vi "Begin.vi"(8 "error in":errorcluster) -> (0 "error out":errorcluster)   [LabVIEW 2019]
doc: "Called before other user functions, this VI is expected to open initial I/O refnums, load in file data, and do all program initialization. Notice that the <B>error out</B> terminal is simply used for data flow. Wiring it to other structures or subVIs ensures that this VI runs first."
uses:
  <vilib>/Rock Robotics/SystemInterfaces/DIO/FPGA_DIOPWMChannel.ctl
  <vilib>/Rock Robotics/WPI/SafetyOutput/WPI_SafetyOutputConfigMenu.ctl
  <vilib>/Rock Robotics/WPI/DriverStation/WPI_DriverStationRobotMode2.ctl
  <vilib>/Rock Robotics/WPI/Joystick/WPI_JoystickDeviceEnum.ctl
  <vilib>/Rock Robotics/SystemInterfaces/AI/FPGA_AIGyroChannel.ctl
  <vilib>/Rock Robotics/SystemInterfaces/DIO/FPGA_DIOChannel.ctl
  <vilib>/Rock Robotics/WPI/Encoder/WPI_EncoderType.ctl
  <vilib>/Rock Robotics/WPI/RobotDrive/WPI_RobotDriveOpen2MotorWithTalon.vi
  Robot Global Data.vi
  <vilib>/Rock Robotics/Network Tables/NT Write String Array.vi
  <vilib>/Rock Robotics/WPI/Gyro/WPI_GyroAnalogOpen.vi
  <vilib>/Rock Robotics/WPI/Counter/WPI_CounterDigitalInputToDigitalSource.vi
panel:
  in  "Tab Control":T1(tab)
  # "Instructions:\nThis should create a path, show the data on the various tabs and optionally write the motor demands and expected results to a file for use on a a robot..\n1) Enter robot data on Robot Data Tab\n2) Define your path definitions.\n3) Define the time increment.  0.020 is chosen since that matches the normal loop time.\n4) Press calculate path.  If a good path was calculated it will be displayed on the Tank Data tab, and the Ready to Execute will indicate execution can begin.\nThe path can be recalculated many times before selecting execute.\n\nTo write to a file.\n5) Select the file name\n6) This example uses \"steps\", sequential numbers for inclusion into a list based autonomous routine.  Including the step number if optional.\n7) This uses command numbers to indicate first, last, and intermediate steps.  This allows some simplification of the execution routine.  It\nalso allows the path to be executed backwards if desired.  The command numbers are changeable.\n8) Press \"Create Command List\".\n\nNotes:\n- PC robot simulataion is disabled in this program.  The code is still there if you want to restore it and try it out.  Use one of the other test programs \nto simulate the path on a PC.\n- The path generation logic doesn't account distribution of speed to the left and right wheels.  As a result the maximum speed can be exceeded.\nIf this happens, but Path Speed > Max light will light and Ready to Execute will not light.  Lower the maximum speed in the Robot Data tab\nand recalulate the path.\n- 2019 playing field size - width: 26 ft 11.25 In = 323.25 in , length: 52 ft 5.25 in = 629.25 in  (I didn't verify this for the 2020 version.)"
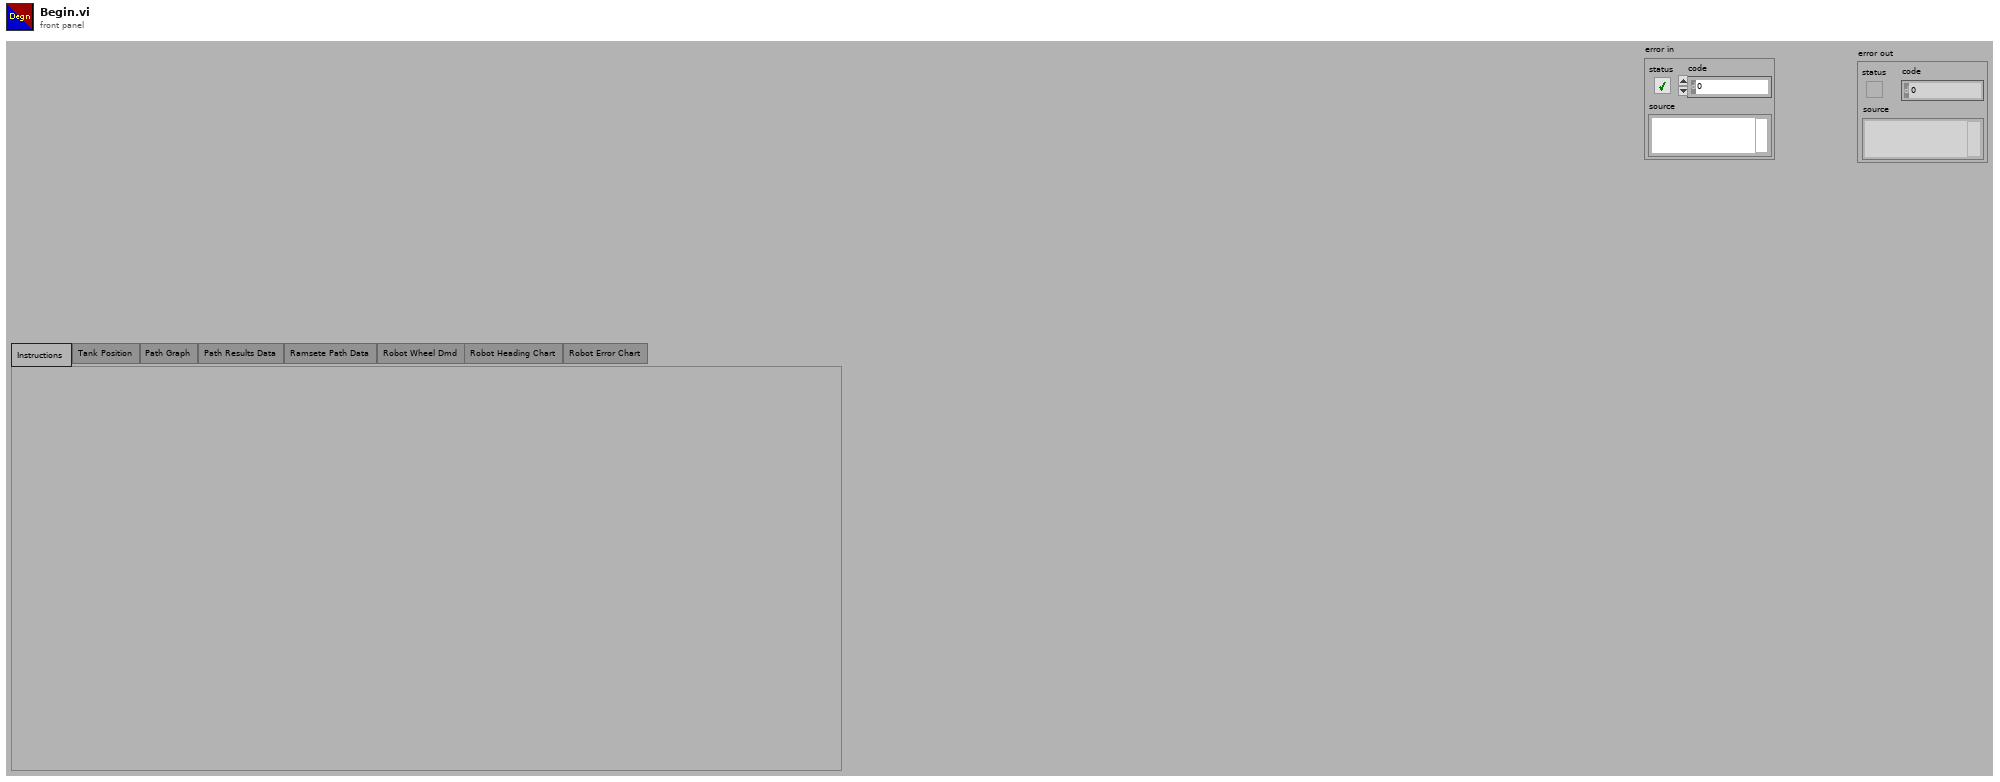
[diagram p1: front panel]
types:
  T1 = enum32{"Instructions", "Tank Position", "Path Graph", "Path Results Data", "Ramsete Path Data", "Robot Wheel Dmd", "Robot Heading Chart", "Robot Error Chart"}
  T2 = typedef "WPI_EncoderType.ctl" = enum16{"1x", "2x", "4x"}
  T3 = typedef "FPGA_DIOChannel.ctl" = enum8{"DIO 0", "DIO 1", "DIO 2", "DIO 3", "DIO 4", "DIO 5", "DIO 6", "DIO 7", "DIO 8", "DIO 9", "DIO MXP 0", "DIO MXP 1", "DIO MXP 2", "DIO MXP 3", "DIO MXP 4", "DIO MXP 5", "DIO MXP 6", "DIO MXP 7", "DIO MXP 8", "DIO MXP 9", "DIO MXP 10", "DIO MXP 11", "DIO MXP 12", "DIO MXP 13", "DIO MXP 14", "DIO MXP 15", "SPI Port CS1", "SPI Port CS2", "SPI Port CS3", "SPI Port MISO", "SPI Port MOSI", "Invalid"}
  T4 = typedef "FPGA_AIGyroChannel.ctl" = enum8{"AI 0", "AI 1", "Invalid"}
  T5 = typedef "WPI_JoystickDeviceEnum.ctl" = enum16{"USB 0", "USB 1", "USB 2", "USB 3", "USB 4", "USB 5"}
  T6 = typedef "WPI_DriverStationRobotMode2.ctl" = enum16{"Autonomous Disabled", "Autonomous Enabled", "Teleop Disabled", "Teleop Enabled", "Disconnected", "Finish", "Test Disabled", "Test Enabled", "Emergency Stopped"}
  T7 = typedef "WPI_SafetyOutputConfigMenu.ctl" = enum16{"Enable", "Disable"}
  T8 = typedef "FPGA_DIOPWMChannel.ctl" = enum8{"PWM 0", "PWM 1", "PWM 2", "PWM 3", "PWM 4", "PWM 5", "PWM 6", "PWM 7", "PWM 8", "PWM 9", "PWM MXP 0", "PWM MXP 1", "PWM MXP 2", "PWM MXP 3", "PWM MXP 4", "PWM MXP 5", "PWM MXP 6", "PWM MXP 7", "PWM MXP 8", "PWM MXP 9", "Invalid"}
  T9 = typedef "WPI_JoystickDevRef.ctl" = cluster{"Device":T5}
  T10 = typedef "WPI_RobotDriveDevRef.ctl" = cluster{"DevStatus":errorcluster, "Motors[]":T11[], "Square Inputs":bool, "Max Output":dbl}
  T11 = typedef "WPI_MotorControlDeviceRef.ctl" = cluster{"DeviceStatus":errorcluster, "Type":T12, "PWM":cluster{"PWM Channel":T8, "DeadBand":T13}, "CAN":cluster{"Device Number":u8, "SetOutput VI Ref":variant, "GetOutput VI Ref":variant, "Enable VI Ref":variant, "Disable VI Ref":variant, "Data":variant}, "Invert":bool, "DIO PWM":cluster{"PWM \"Enable\" Channel":T8, "DIOChannel":T3, "PWM Rate":dbl}}
  T12 = typedef "WPI_MotorControlType.ctl" = enum16{"PWM", "CAN", "DIO PWM"}
  T13 = typedef "WPI_PWMDeadband.ctl" = cluster{"Name":string, "maxPositivePwm":i32, "minPositivePwm":i32, "centerPwm":i32, "maxNegativePwm":i32, "minNegativePwm":i32, "angularRange":u16}
  T14 = typedef "WPI_DigitalInputDevRef.ctl" = cluster{"DevStatus":errorcluster, "DIO Channel":T3}
  T15 = typedef "FPGA_CounterEncoderSourceConvertionLVSourceType.ctl" = cluster{"DevStatus":errorcluster, "AnalogTriggerMode?":bool, "DigitalMode":cluster{"DIO Channel":T16}, "AnalogTriggerMode":cluster{"AnalogTriggerIndex":T17, "OutputType":T18}}
  T16 = typedef "FPGA_DIODigitalSourceChannel.ctl" = enum8{"DIO 0", "DIO 1", "DIO 2", "DIO 3", "DIO 4", "DIO 5", "DIO 6", "DIO 7", "DIO 8", "DIO 9", "DIO MXP 0", "DIO MXP 1", "DIO MXP 2", "DIO MXP 3", "DIO MXP 4", "DIO MXP 5", "DIO MXP 6", "DIO MXP 7", "DIO MXP 8", "DIO MXP 9", "DIO MXP 10", "DIO MXP 11", "DIO MXP 12", "DIO MXP 13", "DIO MXP 14", "DIO MXP 15", "SPI Port CS1", "SPI Port CS2", "SPI Port CS3", "SPI Port MISO", "SPI Port MOSI", "Disabled"}
  T17 = typedef "FPGA_AnalogTriggerIndex.ctl" = enum8{"Trig 0", "Trig 1", "Trig 2", "Trig 3", "Trig 4", "Trig 5", "Trig 6", "Trig 7", "Invalid"}
  T18 = typedef "FPGA_AnalogTriggerOutType.ctl" = enum16{"InWindow", "TriggerState", "Rising", "Falling"}
  T19 = typedef "WPI_EncoderDevRef.ctl" = cluster{"DevStatus":errorcluster, "EncoderIndex":T20, "CounterIndex":T21, "DistancePerCount":dbl, "Decoding Type":T2}
  T20 = typedef "FPGA_EncoderIdx.ctl" = enum8{"Enc 0", "Enc 1", "Enc 2", "Enc 3", "Enc 4", "Enc 5", "Enc 6", "Enc 7", "Invalid"}
  T21 = typedef "FPGA_CounterCtrSystemIndex.ctl" = enum8{"Ctr 0", "Ctr 1", "Ctr 2", "Ctr 3", "Ctr 4", "Ctr 5", "Ctr 6", "Ctr 7", "Invalid"}
  T22 = typedef "WPI_GyroDevRef.ctl" = cluster{"DevStatus":errorcluster, "Analog Channel":T23, "Gain (VoltsPerDegree/Second)":dbl, "Gyro Type":enum16{"Analog", "XRS450"}, "Handle":i32, "SPI Bus":T24, "Device Found":bool, "Sample Rate":dbl, "Calibrate On Open":bool, "Offset":dbl}
  T23 = typedef "FPGA_AIChannel.ctl" = enum8{"AI 0", "AI 1", "AI 2", "AI 3", "AI MXP 0", "AI MXP 1", "AI MXP 2", "AI MXP 3", "Invalid"}
  T24 = typedef "spi_bus.ctl" = enum16{"SPI On-Board, CS0", "SPI On-Board, CS1", "SPI On-Board, CS2", "SPI On-Board, CS3", "SPI MXP", "Invalid"}
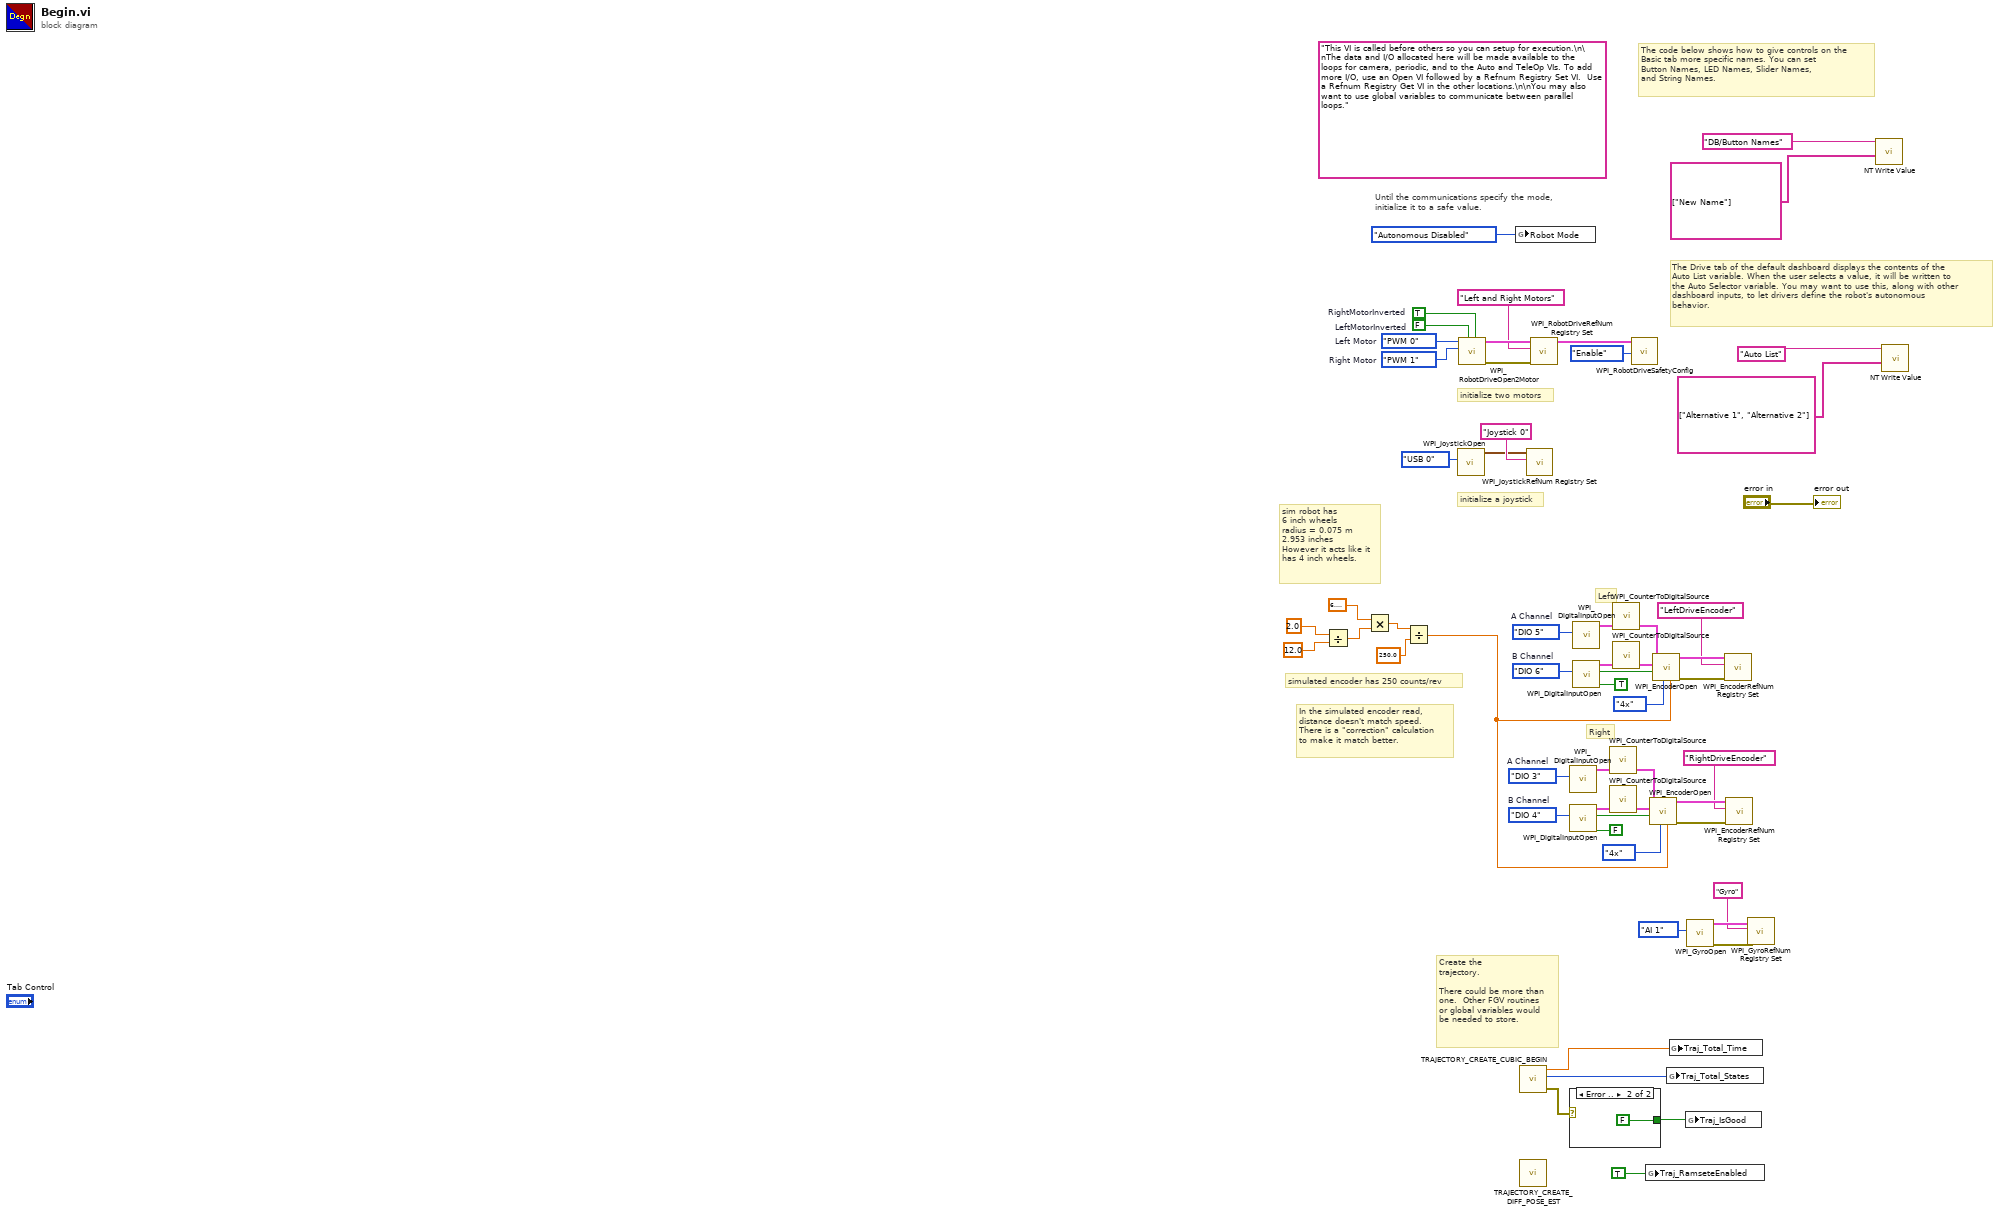
[diagram p0: block diagram]
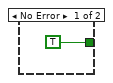
[diagram p2: hidden frame]
diagram:
  w29 = FPGA_DIOChannel."DIO 4"  # B Channel
  w28 = FPGA_DIOChannel."DIO 3"  # A Channel
  w25 = FPGA_DIOChannel."DIO 6"  # B Channel
  w24 = FPGA_DIOChannel."DIO 5"  # A Channel
  (unwired) "This VI is called before others so you can setup for execution.\n\nThe data and I/O allocated here will be made available to the loops for camera, periodic, and to the Auto and TeleOp VIs. To add more I/O, use an Open VI followed by a Refnum Registry Set VI.  Use a Refnum Registry Get VI in the other locations.\n\nYou may also want to use global variables to communicate between parallel loops."
  w50 = FPGA_DIOPWMChannel."PWM 1"  # Right Motor
  w51 = FPGA_DIOPWMChannel."PWM 0"  # Left Motor
  w55 = FALSE  # LeftMotorInverted
  w56 = TRUE  # RightMotorInverted
  # "Create the\ntrajectory.\n\nThere could be more than\none.  Other FGV routines\nor global variables would\nbe needed to store."
  # "In the simulated encoder read,\ndistance doesn't match speed.\nThere is a \"correction\" calculation\nto make it match better."
  # "simulated encoder has 250 counts/rev"
  # "sim robot has\n6 inch wheels\nradius = 0.075 m\n2.953 inches\nHowever it acts like it\nhas 4 inch wheels."
  # "Right"
  # "Left"
  # "The Drive tab of the default dashboard displays the contents of the\nAuto List variable. When the user selects a value, it will be written to\nthe Auto Selector variable. You may want to use this, along with other\ndashboard inputs, to let drivers define the robot's autonomous\nbehavior."
  # "The code below shows how to give controls on the\nBasic tab more specific names. You can set\nButton Names, LED Names, Slider Names,\nand String Names."
  # "initialize a joystick"
  # "Until the communications specify the mode,\ninitialize it to a safe value."
  # "initialize two motors"
  n1 = Divide(x=2.0, y=12.0) -> (x/y=w20:dbl)
  n2 = Multiply(x=6.283185307179586, y=w20) -> (x*y=w21:dbl)
  n3 = Divide(x=w21, y=250.0) -> (x/y=w15:dbl)
  n4 = call <vilib>:"WPI_JoystickOpen.vi"("JoystickDevice"=WPI_JoystickDeviceEnum."USB 0") -> ("JoystickDevRef"=w45:T9)  [unwired: 10 in]
  n5 = call-poly <vilib>:"WPI_RobotDriveOpen2Motor.vi"("Right Motor Inverted"=w56, "Left Motor Inverted"=w55, "Right Motor"=w50, "Left Motor"=w51) -> ("error out"=w52:errorcluster, "RobotDriveDevRef"=w54:T10)  [unwired: 1 in, 5 out]
  n6 = global write "Robot Global Data.vi" "Robot Mode"(WPI_DriverStationRobotMode2."Autonomous Disabled" ("Robot Mode")) -> ()
  n7 = call "TRAJECTORY_CREATE_CUBIC_BEGIN.vi"() -> ("Trajectory \ncalculation \nerror"=w5:errorcluster, "Trajectory Items"=w2:i32, "TotalTImeSecs"=w3:dbl)  [unwired: 9 in]
  n8 = call "TRAJECTORY_CREATE_DIFF_POSE_EST.vi"() -> ()  [unwired: 12 in]
  n9 = call <vilib>:"WPI_JoystickRefNum Registry Set.vi"("refnum name"="Joystick 0", "JoystickDevRef"=w45) -> ()  [unwired: 8 in, 2 out]
  n10 = call <vilib>:"WPI_RobotDriveRefNum Registry Set.vi"("error in (no error)"=w52, "refnum name"="Left and Right Motors", "RobotDriveDevRef"=w54) -> ("RobotDriveDevRef"=w49:T10)  [unwired: 1 in, 7 out]
  n11 = call <vilib>:"WPI_DigitalInputOpen.vi"("DIO Channel"=w28) -> ("DigitalInputDevRef"=w36:T14)  [unwired: 1 in, 9 out]
  n12 = call <vilib>:"WPI_DigitalInputOpen.vi"("DIO Channel"=w29) -> ("DigitalInputDevRef"=w35:T14)  [unwired: 1 in, 9 out]
  n13 = case shown="Error .." w5 {
    tunnel: [TRUE FALSE] -> w4
    frame No Error {
    }
    frame Error {
    }
  }
  n14 = call <vilib>:"WPI_DigitalInputOpen.vi"("DIO Channel"=w24) -> ("DigitalInputDevRef"=w32:T14)  [unwired: 1 in, 9 out]
  n15 = call <vilib>:"WPI_DigitalInputOpen.vi"("DIO Channel"=w25) -> ("DigitalInputDevRef"=w31:T14)  [unwired: 1 in, 9 out]
  n16 = call-poly <vilib>:"WPI_CounterToDigitalSource.vi"("DigitalInputDevRef"=w36) -> ("Digital Source"=w37:T15)  [unwired: 6 out]
  n17 = call-poly <vilib>:"WPI_CounterToDigitalSource.vi"("DigitalInputDevRef"=w35) -> ("Digital Source"=w34:T15)  [unwired: 6 out]
  n18 = call-poly <vilib>:"WPI_CounterToDigitalSource.vi"("DigitalInputDevRef"=w32) -> ("Digital Source"=w33:T15)  [unwired: 6 out]
  n19 = call-poly <vilib>:"WPI_CounterToDigitalSource.vi"("DigitalInputDevRef"=w31) -> ("Digital Source"=w30:T15)  [unwired: 6 out]
  n20 = call <vilib>:"WPI_RobotDriveSafetyConfig.vi"("mode"=WPI_SafetyOutputConfigMenu."Enable", "RobotDriveDevRef"=w49) -> ()  [unwired: 8 in, 2 out]
  n21 = global write "Robot Global Data.vi" "Traj_RamseteEnabled"(TRUE) -> ()
  n22 = call <vilib>:"WPI_EncoderOpen.vi"("DistancePerCount"=w15, "Decoding Type"=WPI_EncoderType."4x", "Invert Direction (False)"=FALSE, "BSource"=w34, "ASource"=w37) -> ("error out"=w11:errorcluster, "EncoderDevRef"=w12:T19)  [unwired: 3 in, 2 out]
  n23 = call <vilib>:"WPI_EncoderOpen.vi"("DistancePerCount"=w15, "Decoding Type"=WPI_EncoderType."4x", "Invert Direction (False)"=TRUE, "BSource"=w30, "ASource"=w33) -> ("error out"=w13:errorcluster, "EncoderDevRef"=w14:T19)  [unwired: 3 in, 2 out]
  n24 = global write "Robot Global Data.vi" "Traj_Total_States"(w2) -> ()
  n25 = global write "Robot Global Data.vi" "Traj_Total_Time"(w3) -> ()
  n26 = global write "Robot Global Data.vi" "Traj_IsGood"(w4) -> ()
  n27 = call-poly <vilib>:"WPI_GyroOpen.vi"("Analog Channel"=FPGA_AIGyroChannel."AI 1") -> ("error out"=w8:errorcluster, "GyroDevRef"=w7:T22)  [unwired: 8 in, 1 out]
  n28 = call <vilib>:"WPI_EncoderRefNum Registry Set.vi"("error in (no error)"=w13, "refnum name"="LeftDriveEncoder", "EncoderDevRef"=w14) -> ()  [unwired: 7 in, 2 out]
  n29 = call <vilib>:"WPI_EncoderRefNum Registry Set.vi"("error in (no error)"=w11, "refnum name"="RightDriveEncoder", "EncoderDevRef"=w12) -> ()  [unwired: 7 in, 2 out]
  n30 = call <vilib>:"WPI_GyroRefNum Registry Set.vi"("error in (no error)"=w8, "refnum name"="Gyro", "GyroDevRef"=w7) -> ()  [unwired: 7 in, 2 out]
  n31 = call-poly <vilib>:"NT Write Value.vi"("String Array"=string[] ["New Name"], "Name"="DB/Button Names") -> ()  [unwired: 9 in, 1 out]
  n32 = call-poly <vilib>:"NT Write Value.vi"("String Array"=string[] ["Alternative 1", "Alternative 2"], "Name"="Auto List") -> ()  [unwired: 9 in, 1 out]
  "error out" <- "error in"
